vi "Get Object Size.vi"(4 "Region":T1, 6 "Version ID":string, 8 "error in (no error)":errorcluster, 9 "Bucket":string, 10 "Object Path":string) -> (0 "error out":errorcluster, 3 "Object Size (bytes)":u64)   [LabVIEW 2015, in "LV Interface for Amazon S3.lvlib"]
doc: "This operation <B>returns Object size</B> (in bytes). <B>Note:</B> To determine object size, the last byte of the object is retreived via a Get Object request."
uses:
  LV Interface for Amazon S3.lvlib
  Typedefs/AMZ_S3_LocationConstraint.ctl
  Typedefs/AMZ_S3_API_GET Object Request Parameters.ctl
  Typedefs/AMZ_S3_API_GET Request Range.ctl
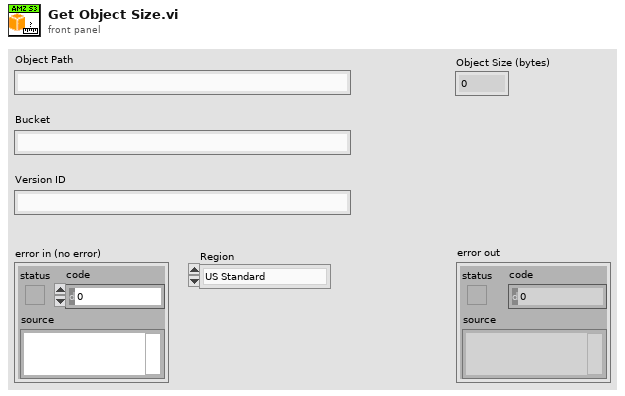
[diagram p1: front panel]
types:
  T1 = typedef "LV Interface for Amazon S3.lvlib/AMZ_S3_LocationConstraint.ctl" = enum16{"US Standard", "us-east-2", "us-west-1", "us-west-2", "ap-northeast-1", "ap-northeast-2", "ap-southeast-1", "ap-southeast-2", "ca-central-1", "eu-central-1", "eu-west-1", "eu-west-2", "sa-east-1"}
  T2 = typedef "LV Interface for Amazon S3.lvlib/AMZ_S3_API_GET Object Request Parameters.ctl" = cluster{"Range":T3, "If Modified Since":timestamp, "If Unmodified Since":timestamp, "Matching ETag":string, "Nonmatching ETag":string}
  T3 = typedef "LV Interface for Amazon S3.lvlib/AMZ_S3_API_GET Request Range.ctl" = cluster{"Start":i64, "Length":i64}
  T4 = typedef "LV Interface for Amazon S3.lvlib/AMZ_S3_API_GETObjectResult.ctl" = cluster{"Content Length (bytes)":u64, "Content Type":string, "ETag":string, "Delete marker":bool, "Version ID":string, "Object Size (bytes)":u64}
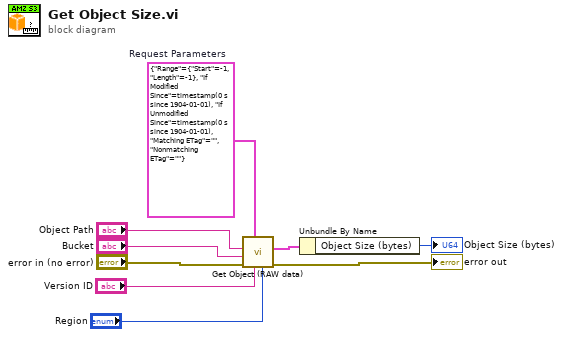
[diagram p0: block diagram]
diagram:
  w9 = T2 {"Range"={"Start"=-1, "Length"=-1}, "If Modified Since"=timestamp(0 s since 1904-01-01), "If Unmodified Since"=timestamp(0 s since 1904-01-01), "Matching ETag"="", "Nonmatching ETag"=""}  # Request Parameters
  n1 = call "Get Object (RAW data).vi"("Region"="Region", "Version ID"="Version ID", "Request Parameters"=w9, "error in (no error)"="error in (no error)", "Bucket"="Bucket", "Object Path"="Object Path") -> ("error out"=→"error out":errorcluster, "GetObjectResult"=w4:T4)  [unwired: 3 in, 1 out]
  n2 = Unbundle By Name(w4) -> ("Object Size (bytes)"=→"Object Size (bytes)":u64)
